vi "Mux8Way16.vi"(0 "c":bool[](array[boolean])=[FALSE, FALSE, FALSE, FALSE, FALSE, FALSE, FALSE, FALSE, FALSE, FALSE, FALSE, FALSE, FALSE, FALSE, FALSE, FALSE], 1 "b":bool[](array[boolean])=[FALSE, FALSE, FALSE, FALSE, FALSE, FALSE, FALSE, FALSE, FALSE, FALSE, FALSE, FALSE, FALSE, FALSE, FALSE, FALSE], 2 "a":bool[](array[boolean])=[FALSE, FALSE, FALSE, FALSE, FALSE, FALSE, FALSE, FALSE, FALSE, FALSE, FALSE, FALSE, FALSE, FALSE, FALSE, FALSE], 5 "d":bool[](array[boolean])=[FALSE, FALSE, FALSE, FALSE, FALSE, FALSE, FALSE, FALSE, FALSE, FALSE, FALSE, FALSE, FALSE, FALSE, FALSE, FALSE], 7 "e":bool[](array[boolean])=[FALSE, FALSE, FALSE, FALSE, FALSE, FALSE, FALSE, FALSE, FALSE, FALSE, FALSE, FALSE, FALSE, FALSE, FALSE, FALSE], 9 "f":bool[](array[boolean])=[FALSE, FALSE, FALSE, FALSE, FALSE, FALSE, FALSE, FALSE, FALSE, FALSE, FALSE, FALSE, FALSE, FALSE, FALSE, FALSE], 11 "g":bool[](array[boolean])=[FALSE, FALSE, FALSE, FALSE, FALSE, FALSE, FALSE, FALSE, FALSE, FALSE, FALSE, FALSE, FALSE, FALSE, FALSE, FALSE], 12 "h":bool[](array[boolean])=[FALSE, FALSE, FALSE, FALSE, FALSE, FALSE, FALSE, FALSE, FALSE, FALSE, FALSE, FALSE, FALSE, FALSE, FALSE, FALSE], 13 "sel":bool[](array[boolean])=[FALSE, FALSE, FALSE]) -> (8 "out":bool[](array[boolean]))   [LabVIEW 2014]
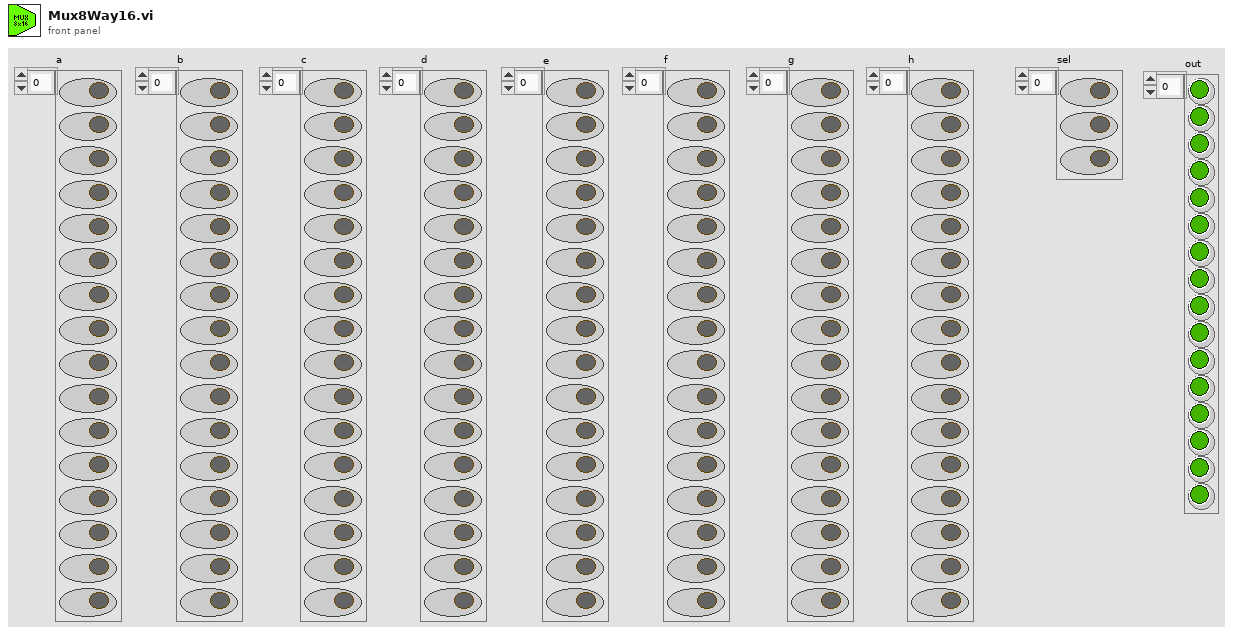
[diagram p1: front panel]
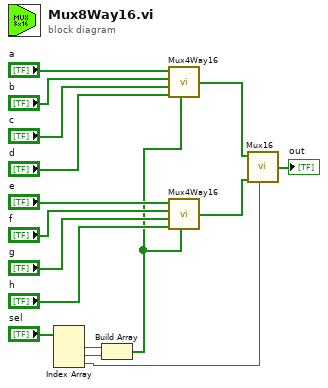
[diagram p0: block diagram]
diagram:
  n1 = Index Array(array="sel") -> (element #1=w3:bool, element #2=w4:bool, element #3=w1:bool)  [unwired: 3 in]
  n2 = Build Array(w3, w4) -> (w2:bool[])
  n3 = call "Mux4Way16.vi"("a"="a", "b"="b", "c"="c", "sel"=w2, "d"="d") -> ("out"=w8:bool[])  [unwired: 3 in]
  n4 = call "Mux4Way16.vi"("a"="e", "b"="f", "c"="g", "sel"=w2, "d"="h") -> ("out"=w7:bool[])  [unwired: 3 in]
  n5 = call "Mux16.vi"("a"=w8, "sel"=w1, "b"=w7) -> ("out"=→"out":bool[])  [unwired: 5 in]
